vi "IRISS_FPGA_IO.vi"() -> ()   [LabVIEW 2016]
doc: "This VI contains a basic quadrature decoder which is reset asynchronously upon clicking the reset button."
uses:
  <vilib>/Platform/TimedLoop/XDataNode/timing_clust.ctl
  <vilib>/Platform/TimedLoop/XDataNode/nitl_modes.ctl
  <vilib>/Platform/TimedLoop/XDataNode/wakeup.ctl
  <vilib>/rvi/Emulation/niFpgaGetClockAttributes.vi
  <vilib>/rvi/Emulation/niFpgaSctlEmulationGetInTimedLoop.vi
  <vilib>/rvi/Emulation/niFpgaEmulationReportErrorSimple.vi
  <vilib>/rvi/eio/common/nirviEmuTemplateMethod_errors.vi
  <vilib>/rvi/Emulation/niFpgaCriticalErrorInLSC.vi
  <vilib>/eio/EIONode/EIONode.xnode
  <vilib>/Platform/TimedLoop/XDataNode/XDataNode.xnode
  <vilib>/Platform/TimedLoop/XDataNode/XDNodeRunTimeDep.lvlib
  Library/KevinLibraryAll/labview/KevLib01.lvlib
  Library/jmslib.lvlib
panel:
  out "Pump Period":i32
  in  "Hydration On/Off (Connector2/DIO28)":bool
  in  "Connector2/DIO7":bool
  in  "Connector2/DIO8":bool
  in  "Connector2/DIO9":bool
  in  "Connector2/DIO10":bool
  in  "PWM1":fxp<+,32,0>
  in  "Period 1 (Ticks)":u32=1000
  in  "Period (Ticks)":u32=2000
  in  "DIR OCT Mot":bool
  in  "INHB OCT Mot":bool
  out "FAULT OCT Mot":bool
  out "Position OCT Mot":i32
  out "JumpBy2Error OCT Mot":i16
  in  "Reset OCT Mot":bool
  in  "OCT Mot DC":fxp<+,32,0>
  in  "Conn0/DIO15 Button 4":bool
  in  "Conn0/DIO12 Button 1":bool
  in  "Conn0/DIO13 Button 2":bool
  out "Home OCT z":bool
  in  "DIR Y":bool
  in  "INHB Y":bool
  out "FAULT Y":bool
  out "Position Y":i32
  out "JumpBy2Error Y":i16
  in  "Reset Y":bool
  in  "Y DC":fxp<+,32,0>
  in  "DIR X":bool
  in  "INHB X":bool
  out "FAULT X":bool
  out "Position X":i32
  out "JumpBy2Error X":i16
  in  "Reset X":bool
  in  "DIR Z":bool
  in  "INHB Z":bool
  out "FAULT Z":bool
  out "Position Z":i32
  out "JumpBy2Error Z":i16
  in  "Reset Z":bool
  in  "Z DC":fxp<+,32,0>
  in  "X DC":fxp<+,32,0>
  out "samples":i32
  out "Current Monitor":u32[](array[numeric])
  out "Raw Data Response (MSB)":bool[](array[boolean])
  out "Home L4":bool
  out "Home L1":bool
  out "Home L2":bool
  out "Home L3":bool
  in  "Positive Direction C1-4":bool
  out "JumpBy2Error C1-4":i16
  out "32 bit Position C1-4":i32
  in  "Reset C1-4":bool
  in  "Positive Direction C1-1":bool
  out "JumpBy2Error C1-1":i16
  out "32 bit Position C1-1":i32
  in  "Reset C1-1":bool
  out "32 bit Position 17":i32
  in  "Reset 17":bool
  in  "Positive Direction 17":bool
  out "JumpBy2Error 17":i16
  out "32 bit Position 16":i32
  in  "Reset 16":bool
  in  "Positive Direction 16":bool
  out "JumpBy2Error 16":i16
  out "32 bit Position 15":i32
  in  "Reset 15":bool
  in  "Positive Direction 15":bool
  out "JumpBy2Error 15":i16
  out "32 bit Position 14":i32
  in  "Reset 14":bool
  in  "Positive Direction 14":bool
  out "JumpBy2Error 14":i16
  out "32 bit Position 13":i32
  in  "Reset 13":bool
  in  "Positive Direction 13":bool
  out "JumpBy2Error 13":i16
  out "32 bit Position 12":i32
  in  "Reset 12":bool
  in  "Positive Direction 12":bool
  out "JumpBy2Error 12":i16
  out "32 bit Position 11":i32
  in  "Reset 11":bool
  in  "Positive Direction 11":bool
  out "JumpBy2Error 11":i16
  out "32 bit Position 10":i32
  in  "Reset 10":bool
  in  "Positive Direction 10":bool
  out "JumpBy2Error 10":i16
  out "32 bit Position 9":i32
  in  "Reset 9":bool
  in  "Positive Direction 9":bool
  out "JumpBy2Error 9":i16
  out "JumpBy2Error 3":i16
  in  "Positive Direction 3":bool
  out "JumpBy2Error 1":i16
  in  "Positive Direction 1":bool
  out "AI":i16[](array[numeric])
  out "32 bit Position 3":i32
  in  "Reset 3":bool
  in  "AO":i16[](array[numeric])=[0, 0, 0, 0, 0, 0, 0, 0]
  out "32 bit Position 1":i32
  in  "Reset 1":bool
  # "Accurus Buttons"
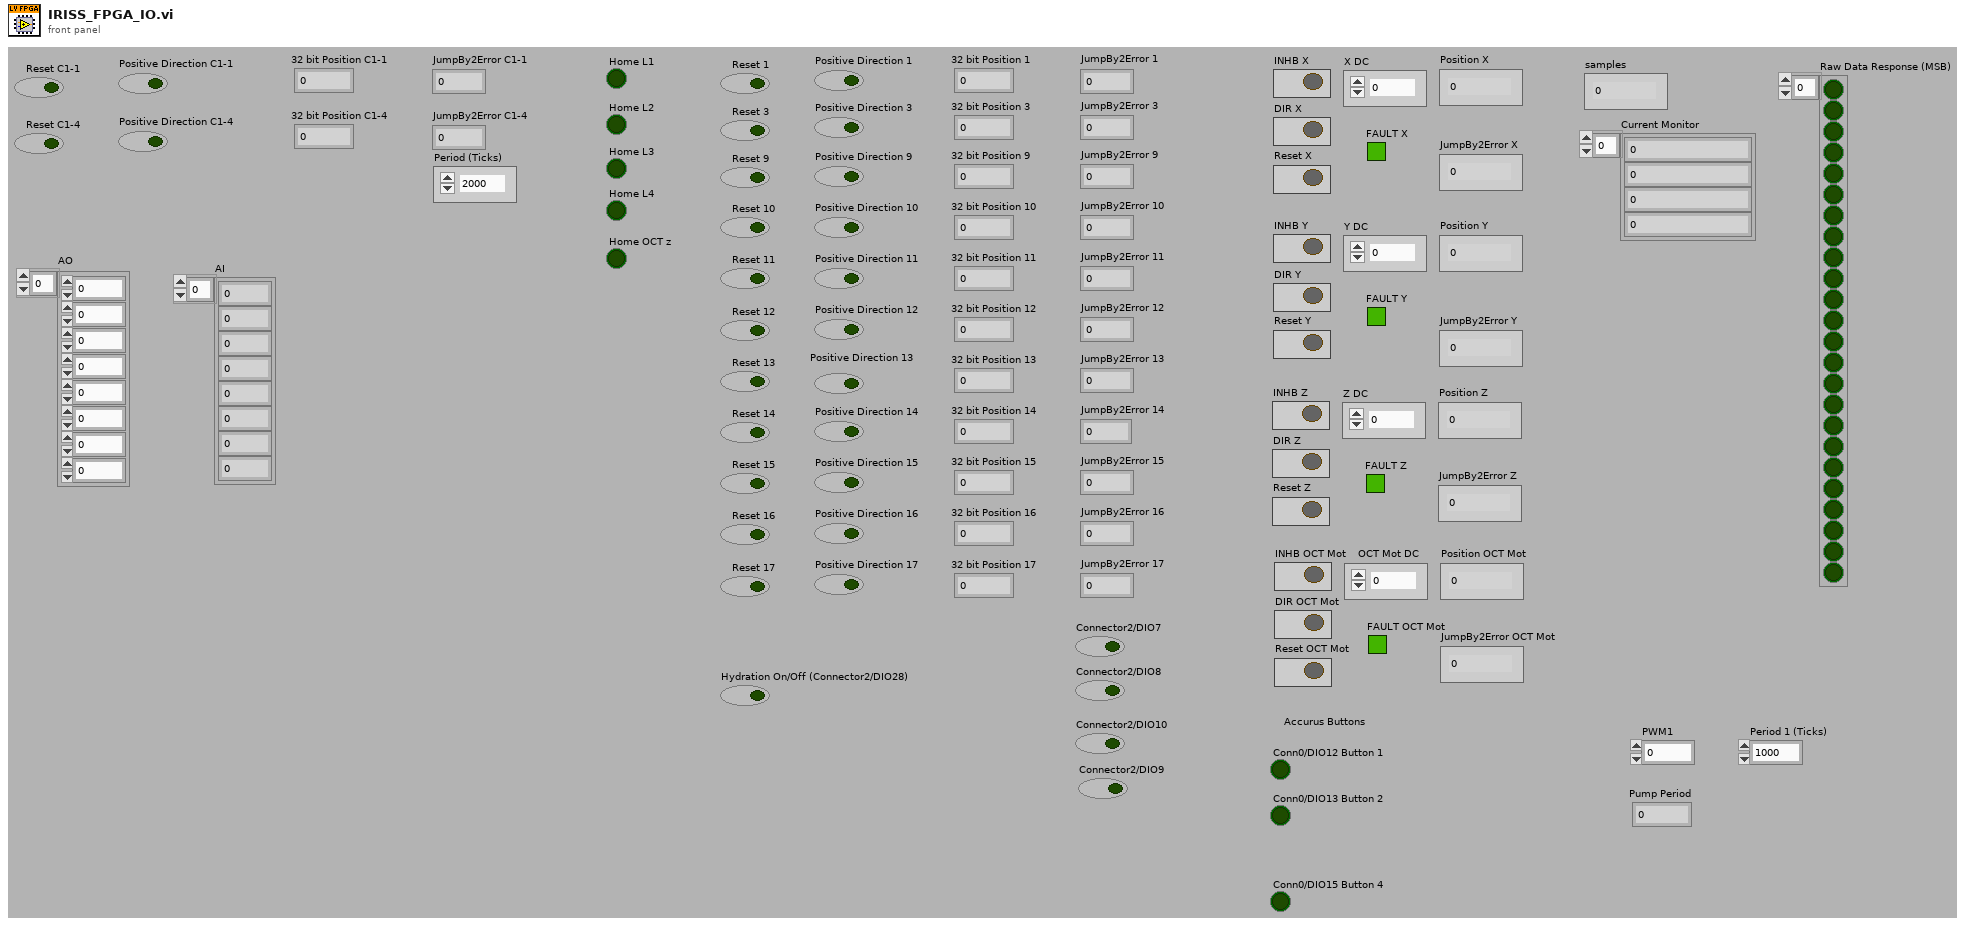
[diagram p1: front panel]
types:
  T1 = typedef "XDNodeRunTimeDep.lvlib/timing_clust.ctl" = cluster{"Expected End [f-1]":u64, "Actual End [f-1]":u64, "Finished Late? [f-1]":bool, "Expected End [i-1]":u64, "Actual End [i-1]":u64, "Finished Late? [i-1]":bool, "Expected Start [i]":u64, "Actual Start [i]":u64, "Expected Start [f]":u64, "Actual Start [f]":u64, "Source Name":string, "Structure Name":string, "Period":i64, "Deadline":i64, "Offset":i64, "Start":i64, "Priority":i32, "Timeout":i32, "Mode":T2, "Wakeup Reason":T3, "Error":errorcluster, "Source Type":string, "Secondary Source Type":string, "Global End Time":u64, "Global Start Time":u64, "Frame Duration":u64, "Iteration Duration":u64, "Assigned CPU":i32, "I/O Scan Engine Mode":u32}
  T2 = typedef "XDNodeRunTimeDep.lvlib/nitl_modes.ctl" = enum32{"No Change", "Process missed periods, maintain original phase", "Discard missed periods, maintain original phase", "Process missed periods, ignore original phase", "Discard missed periods, ignore original phase"}
  T3 = typedef "XDNodeRunTimeDep.lvlib/wakeup.ctl" = enum32{"Normal", "Aborted", "Asynchronous wakeup", "Timing source error", "Timed loop error", "Timeout"}
  T4 = cluster{"PWM In":refnum<k21>, "Direction":refnum<k21>, "Inhibit":refnum<k21>, "Encoder C":refnum<k21>, "Encoder B":refnum<k21>, "Encoder A":refnum<k21>, "Fault":refnum<k21>}
  T5 = cluster{"SCLK":refnum<k21>, "MOSI":refnum<k21>, "MISO":refnum<k21>}
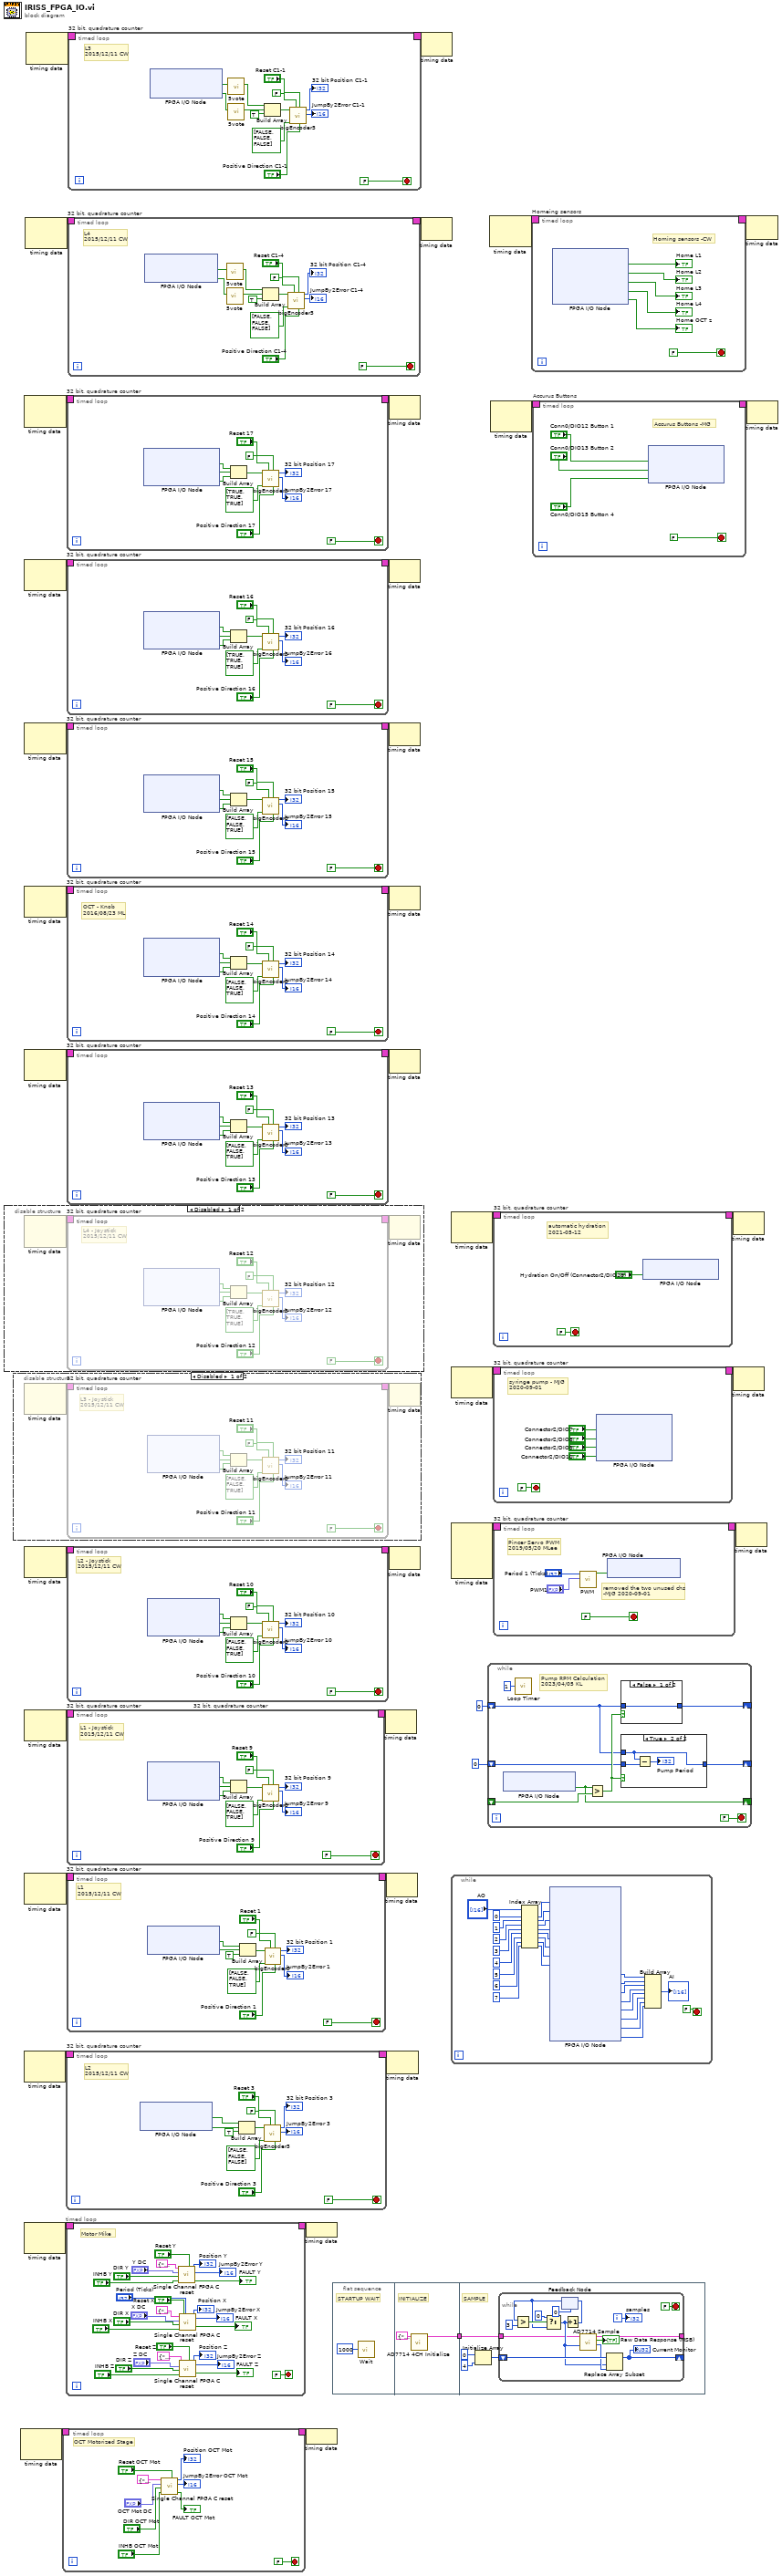
[diagram p0: block diagram]
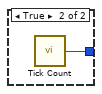
[diagram p3: hidden frame]
diagram:
  n1 = disable-structure shown="Disabled" {
    frame Disabled {
      n2 = node-c288() -> (w41:T1)  [unwired: 2 out]
      n3 = timed-loop "32 bit, quadrature counter" {
        timing-out: [_] -> w40
        timing: w41 -> [_]
        stop <- FALSE stop-if-true
        # "L4 - Joystick\n2015/12/11 CW"
        n4 = xnode "FPGA I/O Node"() -> ("Connector2/DIO9"=w51:bool, "Connector2/DIO10"=w50:bool, "Connector2/DIO11"=w42:bool)  [unwired: 3 in, 3 out]
        n5 = Build Array(w51, w50, w42) -> (w49:bool[])
        n6 = call "bigEncoder3.vi"("Positive Direction"="Positive Direction 12", "ForceReset"="Reset 12", "Allow C Reset?"=FALSE, "Reset Array"=bool[] [TRUE, TRUE, TRUE], "Encoder Array"=w49) -> ("JumpBy2Error"=→"JumpBy2Error 12":i16, "Position"=→"32 bit Position 12":i32)  [unwired: 5 out]
      }
      n7 = node-c288(w40) -> ()  [unwired: 1 out]
    }
    frame Enabled {
    }
  }
  n8 = disable-structure shown="Disabled" {
    frame Disabled {
      n9 = node-c288() -> (w58:T1)  [unwired: 2 out]
      n10 = timed-loop "32 bit, quadrature counter" {
        timing-out: [_] -> w57
        timing: w58 -> [_]
        stop <- FALSE stop-if-true
        # "L3 - Joystick\n2015/12/11 CW"
        n11 = xnode "FPGA I/O Node"() -> ("Connector2/DIO6"=w68:bool, "Connector2/DIO7"=w67:bool, "Connector2/DIO8"=w59:bool)  [unwired: 3 in, 3 out]
        n12 = Build Array(w68, w67, w59) -> (w66:bool[])
        n13 = call "bigEncoder3.vi"("Positive Direction"="Positive Direction 11", "ForceReset"="Reset 11", "Allow C Reset?"=FALSE, "Reset Array"=bool[] [FALSE, FALSE, TRUE], "Encoder Array"=w66) -> ("JumpBy2Error"=→"JumpBy2Error 11":i16, "Position"=→"32 bit Position 11":i32)  [unwired: 5 out]
      }
      n14 = node-c288(w57) -> ()  [unwired: 1 out]
    }
    frame Enabled {
    }
  }
  n15 = node-c288() -> (w12:T1)  [unwired: 2 in]
  n16 = node-c288() -> (w37:T1)  [unwired: 2 out]
  n17 = node-c288() -> (w17:T1)  [unwired: 2 in]
  n18 = node-c288() -> (w25:T1)  [unwired: 2 out]
  n19 = node-c288() -> (w27:T1)  [unwired: 2 out]
  n20 = node-c288() -> (w29:T1)  [unwired: 2 out]
  n21 = node-c288() -> (w31:T1)  [unwired: 2 out]
  n22 = node-c288() -> (w33:T1)  [unwired: 2 out]
  n23 = node-c288() -> (w6:T1)  [unwired: 2 out]
  n24 = node-c288() -> (w35:T1)  [unwired: 2 out]
  n25 = node-c288() -> (w38:T1)  [unwired: 2 out]
  n26 = node-c288() -> (w21:T1)  [unwired: 2 out]
  n27 = node-c288() -> (w23:T1)  [unwired: 2 out]
  n28 = timed-loop {
    timing: w12 -> [_]
    timing-out: [_] -> w11
    stop <- FALSE stop-if-true
    # "OCT Motorized Stage"
    n29 = call "Single Channel FPGA C reset.vi"("Reset"="Reset OCT Mot", "INHB"="INHB OCT Mot", "DIR"="DIR OCT Mot", "Duty"="OCT Mot DC", "IO Channels"=T4 {"PWM In"="Connector1/DIO7", "Direction"="Connector1/DIO8", "Inhibit"="Connector1/DIO9", "Encoder C"="Connector1/DIO10", "Encoder B"="Connector1/DIO11", "Encoder A"="Connector1/DIO12", "Fault"="Connector1/DIO13"}) -> ("FAULT"=→"FAULT OCT Mot":bool, "JumpBy2Error"=→"JumpBy2Error OCT Mot":i16, "Position"=→"Position OCT Mot":i32)  [unwired: 4 in]
  }
  n30 = timed-loop "32 bit, quadrature counter" {
    timing-out: [_] -> w36
    timing: w37 -> [_]
    stop <- FALSE stop-if-true
    # "L2\n2015/12/11 CW"
    n31 = xnode "FPGA I/O Node"() -> ("Connector0/DIO2"=w88:bool, "Connector0/DIO3"=w87:bool)  [unwired: 2 in, 2 out]
    n32 = Build Array(w88, w87, TRUE ("element")) -> (w94:bool[])
    n33 = call "bigEncoder3.vi"("Positive Direction"="Positive Direction 3", "ForceReset"="Reset 3", "Allow C Reset?"=FALSE, "Reset Array"=bool[] [FALSE, FALSE, FALSE], "Encoder Array"=w94) -> ("JumpBy2Error"=→"JumpBy2Error 3":i16, "Position"=→"32 bit Position 3":i32)  [unwired: 5 out]
  }
  n34 = timed-loop {
    timing: w17 -> [_]
    timing-out: [_] -> w16
    stop <- FALSE stop-if-true
    # "Motor Mike"
    n35 = call "Single Channel FPGA C reset.vi"("Reset"="Reset Y", "INHB"="INHB Y", "DIR"="DIR Y", "Duty"="Y DC", "IO Channels"=T4 {"PWM In"="Connector1/DIO1", "Direction"="Connector1/DIO2", "Inhibit"="Connector1/DIO3", "Encoder C"="Connector1/DIO4", "Encoder B"="Connector1/DIO5", "Encoder A"="Connector1/DIO6", "Fault"="Connector1/DIO0"}) -> ("FAULT"=→"FAULT Y":bool, "JumpBy2Error"=→"JumpBy2Error Y":i16, "Position"=→"Position Y":i32)  [unwired: 4 in]
    n36 = call "Single Channel FPGA C reset.vi"("Reset"="Reset X", "Period (Ticks)"="Period (Ticks)", "INHB"="INHB X", "DIR"="DIR X", "Duty"="X DC", "IO Channels"=T4 {"PWM In"="Connector1/DIO20", "Direction"="Connector1/DIO21", "Inhibit"="Connector1/DIO22", "Encoder C"="Connector1/DIO23", "Encoder B"="Connector1/DIO24", "Encoder A"="Connector1/DIO25", "Fault"="Connector1/DIO27"}) -> ("FAULT"=→"FAULT X":bool, "JumpBy2Error"=→"JumpBy2Error X":i16, "Position"=→"Position X":i32)  [unwired: 3 in]
    n37 = call "Single Channel FPGA C reset.vi"("Reset"="Reset Z", "INHB"="INHB Z", "DIR"="DIR Z", "Duty"="Z DC", "IO Channels"=T4 {"PWM In"="Connector1/DIO14", "Direction"="Connector1/DIO15", "Inhibit"="Connector1/DIO16", "Encoder C"="Connector1/DIO17", "Encoder B"="Connector1/DIO18", "Encoder A"="Connector1/DIO19", "Fault"="Connector1/DIO26"}) -> ("FAULT"=→"FAULT Z":bool, "JumpBy2Error"=→"JumpBy2Error Z":i16, "Position"=→"Position Z":i32)  [unwired: 4 in]
  }
  n38 = timed-loop "32 bit, quadrature counter" {
    timing-out: [_] -> w24
    timing: w25 -> [_]
    stop <- FALSE stop-if-true
    n39 = xnode "FPGA I/O Node"() -> ("Connector2/DIO24"=w135:bool, "Connector2/DIO25"=w134:bool, "Connector2/DIO26"=w126:bool)  [unwired: 3 in, 3 out]
    n40 = Build Array(w135, w134, w126) -> (w133:bool[])
    n41 = call "bigEncoder3.vi"("Positive Direction"="Positive Direction 17", "ForceReset"="Reset 17", "Allow C Reset?"=FALSE, "Reset Array"=bool[] [TRUE, TRUE, TRUE], "Encoder Array"=w133) -> ("JumpBy2Error"=→"JumpBy2Error 17":i16, "Position"=→"32 bit Position 17":i32)  [unwired: 5 out]
  }
  n42 = timed-loop "32 bit, quadrature counter" {
    timing-out: [_] -> w26
    timing: w27 -> [_]
    stop <- FALSE stop-if-true
    n43 = xnode "FPGA I/O Node"() -> ("Connector2/DIO21"=w148:bool, "Connector2/DIO22"=w147:bool, "Connector2/DIO23"=w139:bool)  [unwired: 3 in, 3 out]
    n44 = Build Array(w148, w147, w139) -> (w146:bool[])
    n45 = call "bigEncoder3.vi"("Positive Direction"="Positive Direction 16", "ForceReset"="Reset 16", "Allow C Reset?"=FALSE, "Reset Array"=bool[] [TRUE, TRUE, TRUE], "Encoder Array"=w146) -> ("JumpBy2Error"=→"JumpBy2Error 16":i16, "Position"=→"32 bit Position 16":i32)  [unwired: 5 out]
  }
  n46 = timed-loop "32 bit, quadrature counter" {
    timing-out: [_] -> w28
    timing: w29 -> [_]
    stop <- FALSE stop-if-true
    n47 = xnode "FPGA I/O Node"() -> ("Connector2/DIO18"=w161:bool, "Connector2/DIO19"=w160:bool, "Connector2/DIO20"=w152:bool)  [unwired: 3 in, 3 out]
    n48 = Build Array(w161, w160, w152) -> (w159:bool[])
    n49 = call "bigEncoder3.vi"("Positive Direction"="Positive Direction 15", "ForceReset"="Reset 15", "Allow C Reset?"=FALSE, "Reset Array"=bool[] [FALSE, FALSE, TRUE], "Encoder Array"=w159) -> ("JumpBy2Error"=→"JumpBy2Error 15":i16, "Position"=→"32 bit Position 15":i32)  [unwired: 5 out]
  }
  n50 = timed-loop "32 bit, quadrature counter" {
    timing-out: [_] -> w30
    timing: w31 -> [_]
    stop <- FALSE stop-if-true
    # "OCT - Knob\n2016/08/23 ML"
    n51 = xnode "FPGA I/O Node"() -> ("Connector2/DIO15"=w174:bool, "Connector2/DIO16"=w173:bool, "Connector2/DIO17"=w165:bool)  [unwired: 3 in, 3 out]
    n52 = Build Array(w174, w173, w165) -> (w172:bool[])
    n53 = call "bigEncoder3.vi"("Positive Direction"="Positive Direction 14", "ForceReset"="Reset 14", "Allow C Reset?"=FALSE, "Reset Array"=bool[] [FALSE, FALSE, TRUE], "Encoder Array"=w172) -> ("JumpBy2Error"=→"JumpBy2Error 14":i16, "Position"=→"32 bit Position 14":i32)  [unwired: 5 out]
  }
  n54 = timed-loop "32 bit, quadrature counter" {
    timing-out: [_] -> w32
    timing: w33 -> [_]
    stop <- FALSE stop-if-true
    n55 = xnode "FPGA I/O Node"() -> ("Connector2/DIO12"=w187:bool, "Connector2/DIO13"=w186:bool, "Connector2/DIO14"=w178:bool)  [unwired: 3 in, 3 out]
    n56 = Build Array(w187, w186, w178) -> (w185:bool[])
    n57 = call "bigEncoder3.vi"("Positive Direction"="Positive Direction 13", "ForceReset"="Reset 13", "Allow C Reset?"=FALSE, "Reset Array"=bool[] [FALSE, FALSE, TRUE], "Encoder Array"=w185) -> ("JumpBy2Error"=→"JumpBy2Error 13":i16, "Position"=→"32 bit Position 13":i32)  [unwired: 5 out]
  }
  n58 = timed-loop "32 bit, quadrature counter" {
    timing-out: [_] -> w5
    timing: w6 -> [_]
    stop <- FALSE stop-if-true
    # "L2 - Joystick\n2015/12/11 CW"
    n59 = xnode "FPGA I/O Node"() -> ("Connector2/DIO3"=w200:bool, "Connector2/DIO4"=w199:bool, "Connector2/DIO5"=w191:bool)  [unwired: 3 in, 3 out]
    n60 = Build Array(w200, w199, w191) -> (w198:bool[])
    n61 = call "bigEncoder3.vi"("Positive Direction"="Positive Direction 10", "ForceReset"="Reset 10", "Allow C Reset?"=FALSE, "Reset Array"=bool[] [FALSE, FALSE, TRUE], "Encoder Array"=w198) -> ("JumpBy2Error"=→"JumpBy2Error 10":i16, "Position"=→"32 bit Position 10":i32)  [unwired: 5 out]
  }
  n62 = timed-loop "32 bit, quadrature counter" {
    timing-out: [_] -> w34
    timing: w35 -> [_]
    stop <- FALSE stop-if-true
    # "L1 - Joystick\n2015/12/11 CW"
    n63 = xnode "FPGA I/O Node"() -> ("Connector2/DIO0"=w213:bool, "Connector2/DIO1"=w212:bool, "Connector2/DIO2"=w204:bool)  [unwired: 3 in, 3 out]
    n64 = Build Array(w213, w212, w204) -> (w211:bool[])
    n65 = call "bigEncoder3.vi"("Positive Direction"="Positive Direction 9", "ForceReset"="Reset 9", "Allow C Reset?"=FALSE, "Reset Array"=bool[] [FALSE, FALSE, TRUE], "Encoder Array"=w211) -> ("JumpBy2Error"=→"JumpBy2Error 9":i16, "Position"=→"32 bit Position 9":i32)  [unwired: 5 out]
  }
  n66 = timed-loop "32 bit, quadrature counter" {
    timing-out: [_] -> w39
    timing: w38 -> [_]
    stop <- FALSE stop-if-true
    # "L1\n2015/12/11 CW"
    n67 = xnode "FPGA I/O Node"() -> ("Connector0/DIO0"=w226:bool, "Connector0/DIO1"=w225:bool)  [unwired: 2 in, 2 out]
    n68 = Build Array(w226, w225, TRUE ("element")) -> (w224:bool[])
    n69 = call "bigEncoder3.vi"("Positive Direction"="Positive Direction 1", "ForceReset"="Reset 1", "Allow C Reset?"=FALSE, "Reset Array"=bool[] [FALSE, FALSE, TRUE], "Encoder Array"=w224) -> ("JumpBy2Error"=→"JumpBy2Error 1":i16, "Position"=→"32 bit Position 1":i32)  [unwired: 5 out]
  }
  n70 = timed-loop "32 bit, quadrature counter" {
    timing-out: [_] -> w20
    timing: w21 -> [_]
    stop <- FALSE stop-if-true
    # "L4\n2015/12/11 CW"
    n71 = xnode "FPGA I/O Node"() -> ("Connector0/DIO6"=w233:bool, "Connector0/DIO7"=w232:bool)  [unwired: 2 in, 2 out]
    n72 = call "5vote.vi"("Input"=w233) -> ("vote5"=w230:bool)  [unwired: 10 in]
    n73 = call "5vote.vi"("Input"=w232) -> ("vote5"=w231:bool)  [unwired: 10 in]
    n74 = Build Array(w230, w231, TRUE ("element")) -> (w241:bool[])
    n75 = call "bigEncoder3.vi"("Positive Direction"="Positive Direction C1-4", "ForceReset"="Reset C1-4", "Allow C Reset?"=FALSE, "Reset Array"=bool[] [FALSE, FALSE, FALSE], "Encoder Array"=w241) -> ("JumpBy2Error"=→"JumpBy2Error C1-4":i16, "Position"=→"32 bit Position C1-4":i32)  [unwired: 5 out]
  }
  n76 = timed-loop "32 bit, quadrature counter" {
    timing-out: [_] -> w22
    timing: w23 -> [_]
    stop <- FALSE stop-if-true
    # "L3\n2015/12/11 CW"
    n77 = xnode "FPGA I/O Node"() -> ("Connector0/DIO4"=w248:bool, "Connector0/DIO5"=w247:bool)  [unwired: 2 in, 2 out]
    n78 = call "5vote.vi"("Input"=w248) -> ("vote5"=w245:bool)  [unwired: 10 in]
    n79 = call "5vote.vi"("Input"=w247) -> ("vote5"=w246:bool)  [unwired: 10 in]
    n80 = Build Array(w245, w246, TRUE ("element")) -> (w256:bool[])
    n81 = call "bigEncoder3.vi"("Positive Direction"="Positive Direction C1-1", "ForceReset"="Reset C1-1", "Allow C Reset?"=FALSE, "Reset Array"=bool[] [FALSE, FALSE, FALSE], "Encoder Array"=w256) -> ("JumpBy2Error"=→"JumpBy2Error C1-1":i16, "Position"=→"32 bit Position C1-1":i32)  [unwired: 5 out]
  }
  n82 = node-c288(w16) -> ()
  n83 = node-c288(w11) -> ()
  n84 = flat-sequence {
    tunnel: [w261] -> w15
    tunnel: w15 -> [w263]
    frame #0 {
      # "STARTUP WAIT"
      n85 = call "Wait"("Count(uSec)"=u32 1000) -> ()  [unwired: 1 out]
    }
    frame #1 {
      # "INITIALIZE"
      n86 = call "AD7714 4CH Initialize.vi"("I/O Cluster In"=T5 {"SCLK"="Connector1/DIO29", "MOSI"="Connector1/DIO35", "MISO"="Connector1/DIO31"}) -> ("I/O Cluster Out"=w261:T5)  [unwired: 10 in]
    }
    frame #2 {
      # "SAMPLE"
      n87 = Initialize Array(u32 0, 4 ("dimension size")) -> (w264:u32[])
      n88 = while {
        shift-right: [w272] -> _
        shift-left: w264 -> [w273]
        tunnel: w263 -> [w269]
        tunnel: [w268] -> _
        i -> [w280]
        stop <- FALSE stop-if-true
        n89 = feedback #1(i16 0) -> (w276:i16)
        n90 = Greater?(x=w276, y=i16 3) -> (0:w277:bool)
        n91 = Select(t=i16 0, s=w277, f=w276) -> (s? t:f=w270:i16)
        n92 = Increment(x=w270) -> (x+1=w274:i16)
        n93 = feedback-in #1(w274) -> ()
        n94 = call "AD7714 Sample.vi"("Channel"=w270, "I/O Cluster In"=w269) -> ("Data"=w271:u32, "Raw Data Response (MSB)"=→"Raw Data Response (MSB)":bool[], "I/O Cluster Out"=w268:T5)  [unwired: 7 in]
        n95 = Replace Array Subset(array=w273, new element=w271, index=w270) -> (w272:u32[])
        "Current Monitor" <- w272
        "samples" <- w280
      }
    }
  }
  n96 = node-c288(w34) -> ()  [unwired: 1 out]
  n97 = node-c288(w39) -> ()  [unwired: 1 out]
  n98 = node-c288(w36) -> ()  [unwired: 1 out]
  n99 = node-c288(w24) -> ()  [unwired: 1 out]
  n100 = node-c288(w26) -> ()  [unwired: 1 out]
  n101 = node-c288(w28) -> ()  [unwired: 1 out]
  n102 = node-c288(w30) -> ()  [unwired: 1 out]
  n103 = node-c288(w32) -> ()  [unwired: 1 out]
  n104 = node-c288(w5) -> ()  [unwired: 1 out]
  n105 = node-c288(w20) -> ()  [unwired: 1 out]
  n106 = node-c288(w22) -> ()  [unwired: 1 out]
  n107 = node-c288() -> (w4:T1)  [unwired: 2 out]
  n108 = node-c288() -> (w8:T1)  [unwired: 2 out]
  n109 = node-c288() -> (w10:T1)  [unwired: 4 in, 1 out]
  n110 = while {
    stop <- FALSE stop-if-true
    n111 = Index Array(array="AO", index #1=0 ("index"), index #2=1 ("index"), index #3=2 ("index"), index #4=3 ("index"), index #5=4 ("index"), index #6=5 ("index"), index #7=6 ("index"), index #8=7 ("index")) -> (element #1=w299:i16, element #2=w298:i16, element #3=w297:i16, element #4=w296:i16, element #5=w295:i16, element #6=w294:i16, element #7=w293:i16, element #8=w292:i16)
    n112 = xnode "FPGA I/O Node"("Connector0/AO0"=w299, "Connector0/AO1"=w298, "Connector0/AO2"=w297, "Connector0/AO3"=w296, "Connector0/AO4"=w295, "Connector0/AO5"=w294, "Connector0/AO6"=w293, "Connector0/AO7"=w292) -> ("Connector0/AI0"=w290:i16, "Connector0/AI1"=w289:i16, "Connector0/AI2"=w287:i16, "Connector0/AI3"=w286:i16, "Connector0/AI4"=w285:i16, "Connector0/AI5"=w284:i16, "Connector0/AI6"=w283:i16, "Connector0/AI7"=w282:i16)  [unwired: 16 in, 16 out]
    n113 = Build Array(w290, w289, w287, w286, w285, w284, w283, w282) -> (→"AI":i16[])
  }
  n114 = while {
    shift-right: [w315] -> _
    shift-left: i16 0 -> [w311]
    shift-right: [w310] -> _
    shift-left: i16 0 -> [w312]
    shift-right: [w314] -> _
    shift-left: _ -> [w316]
    stop <- FALSE stop-if-true
    # "Pump RPM Calculation\n2023/04/05 KL"
    n115 = xnode "FPGA I/O Node"() -> ("Connector2/DIO0"=w314:bool)  [unwired: 1 in, 1 out]
    n116 = call "Loop Timer"("Count(uSec)"=u32 1) -> ()  [unwired: 1 out]
    n117 = Greater?(x=w314, y=w316) -> (0:w313:bool)
    n118 = case shown="False" w313 {
      tunnel: w311 -> [w322 _]
      tunnel: [w322 w323] -> w315
      frame False {
      }
      frame True {
        n119 = call "Tick Count"() -> ("Tick Count(uSec)"=w323:u32)
      }
    }
    n120 = case shown="True" w313 {
      tunnel: w312 -> [w318 w321]
      tunnel: w311 -> [_ w320]
      tunnel: [w318 w320] -> w310
      frame False {
      }
      frame True {
        n121 = Subtract(x=w320, y=w321) -> (x-y=→"Pump Period":u32)
      }
    }
  }
  n122 = node-c288() -> (w19:T1)  [unwired: 2 out]
  n123 = node-c288() -> (w14:T1)  [unwired: 2 out]
  n124 = timed-loop "32 bit, quadrature counter" {
    timing-out: [_] -> w3
    timing: w4 -> [_]
    stop <- FALSE stop-if-true
    # "automatic hydration \n2021-05-12"
    n125 = xnode "FPGA I/O Node"("Connector2/DIO28"="Hydration On/Off (Connector2/DIO28)") -> ()  [unwired: 1 in, 1 out]
  }
  n126 = timed-loop "32 bit, quadrature counter" {
    timing-out: [_] -> w7
    timing: w8 -> [_]
    stop <- FALSE stop-if-true
    # "syringe pump - MJG \n2020-09-01"
    n127 = xnode "FPGA I/O Node"("Connector2/DIO7"="Connector2/DIO7", "Connector2/DIO8"="Connector2/DIO8", "Connector2/DIO9"="Connector2/DIO9", "Connector2/DIO10"="Connector2/DIO10") -> ()  [unwired: 4 in, 4 out]
  }
  n128 = timed-loop "32 bit, quadrature counter" {
    timing-out: [_] -> w9
    timing: w10 -> [_]
    stop <- FALSE stop-if-true
    # "removed the two unused chs\n-MJG 2020-09-01"
    # "Pincer Servo PWM\n2019/05/20 MLee"
    n129 = call "PWM.vi"("Duty Cycle"="PWM1", "Period (Ticks)"="Period 1 (Ticks)") -> ("PWM Out"=w337:bool)  [unwired: 8 in, 1 out]
    n130 = xnode "FPGA I/O Node"("Connector2/DIO6"=w337) -> ()  [unwired: 1 in, 1 out]
  }
  n131 = timed-loop "Homeing sensors" {
    timing-out: [_] -> w18
    timing: w19 -> [_]
    stop <- FALSE stop-if-true
    # "Homing sensors -CW"
    n132 = xnode "FPGA I/O Node"() -> ("Connector0/DIO8"=→"Home L1":bool, "Connector0/DIO9"=→"Home L2":bool, "Connector0/DIO10"=→"Home L3":bool, "Connector0/DIO11"=→"Home L4":bool, "Connector0/DIO14"=→"Home OCT z":bool)  [unwired: 5 in, 5 out]
  }
  n133 = timed-loop "Accurus Buttons" {
    timing-out: [_] -> w13
    timing: w14 -> [_]
    stop <- FALSE stop-if-true
    # "Accurus Buttons -MG"
    n134 = xnode "FPGA I/O Node"("Connector0/DIO12"="Conn0/DIO12 Button 1", "Connector0/DIO13"="Conn0/DIO13 Button 2", "Connector0/DIO15"="Conn0/DIO15 Button 4") -> ()  [unwired: 3 in, 3 out]
  }
  n135 = node-c288(w3) -> ()  [unwired: 1 out]
  n136 = node-c288(w7) -> ()  [unwired: 1 out]
  n137 = node-c288(w9) -> ()  [unwired: 1 out]
  n138 = node-c288(w18) -> ()  [unwired: 1 out]
  n139 = node-c288(w13) -> ()  [unwired: 1 out]
